vi "Make.vi"(8 "error in (no error)":errorcluster, 11 "Electrical in":refnum<class "Petrol.lvclass">) -> (0 "error out":errorcluster, 3 "Electrical out":refnum<class "Petrol.lvclass">)   [LabVIEW 2014, in "Petrol.lvclass"]
uses:
  Petrol.lvclass
  Paint/Paint.lvclass
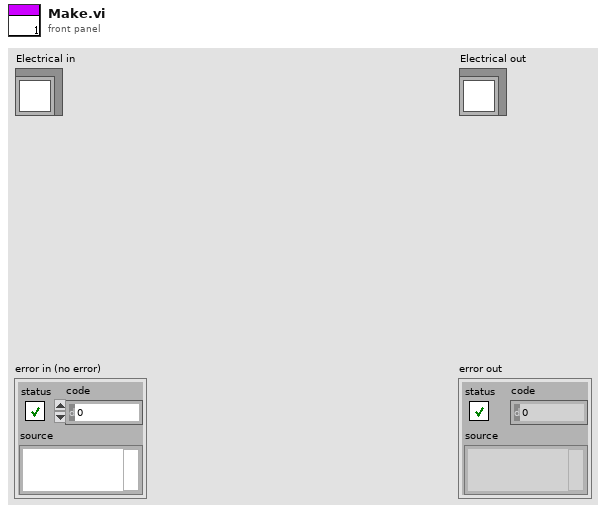
[diagram p1: front panel]
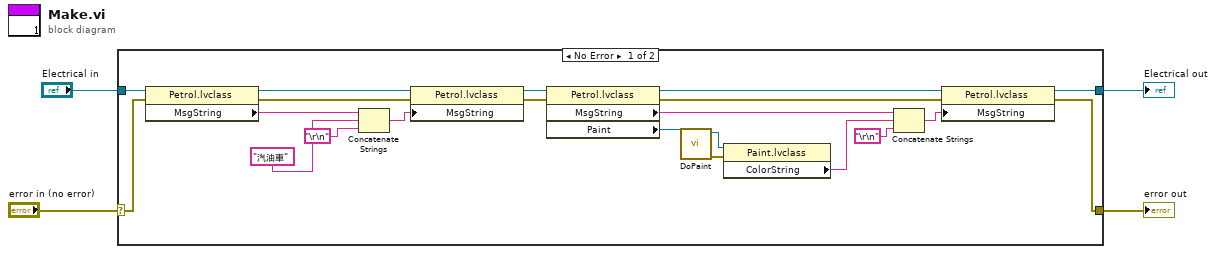
[diagram p0: block diagram]
diagram:
  n1 = case shown="No Error" "error in (no error)" {
    selector: "error in (no error)" -> [w25 w27]
    tunnel: [w14 w27] -> w4
    tunnel: [w12 w26] -> w3
    tunnel: "Electrical in" -> [w23 w26]
    frame No Error {
      n2 = property class="Petrol.lvclass"(reference=w23, error in=w25) -> (reference out=w21:refnum<class "Petrol.lvclass">, error out=w24:errorcluster, "MsgString"=w20:string)
      n3 = Concatenate Strings(w20, "汽油車", "\r\n") -> (w19:string)
      n4 = property class="Petrol.lvclass"(reference=w21, error in=w24, "MsgString"=w19) -> (reference out=w15:refnum<class "Petrol.lvclass">, error out=w22:errorcluster)
      n5 = property class="Petrol.lvclass"(reference=w15, error in=w22) -> (reference out=w13:refnum<class "Petrol.lvclass">, error out=w16:errorcluster, "MsgString"=w10:string, "Paint"=w8:refnum<class "Paint.lvclass">)
      n6 = call-dynamic "DoPaint.vi"("Paint in"=w8) -> ("error out"=w6:errorcluster, "Paint out"=w7:refnum<class "Paint.lvclass">)  [unwired: 9 in]
      n7 = property class="Paint.lvclass"(reference=w7, error in=w6) -> ("ColorString"=w5:string)  [unwired: 2 out]
      n8 = Concatenate Strings(w10, w5, "\r\n") -> (w9:string)
      n9 = property class="Petrol.lvclass"(reference=w13, error in=w16, "MsgString"=w9) -> (reference out=w12:refnum<class "Petrol.lvclass">, error out=w14:errorcluster)
    }
    frame Error {
    }
  }
  "error out" <- w4
  "Electrical out" <- w3
